vi "Enqueue with Error.vi"(8 "error in (no error)":errorcluster, 10 "Command to Queue":string, 11 "queue in":refnum<queue>) -> (0 "error out":errorcluster, 3 "queue out":refnum<queue>)   [LabVIEW 2010]
doc: "This VI enqueues a command (string) into the input queue. In addition, if any errors are present on the error cluster, the Error state is queued before the input command to be executed in the Error case. Once the error state is queued, the error cluster is cleared and normal operation continues.\n\nInputs:\nqueue in - input queue reference (string queue)\ncommand to queue - command/state to queue (string)\nerror in - error input cluster\n\nOutputs:\nqueue out - referece to input queue (dup)\nerror out - error output cluster"
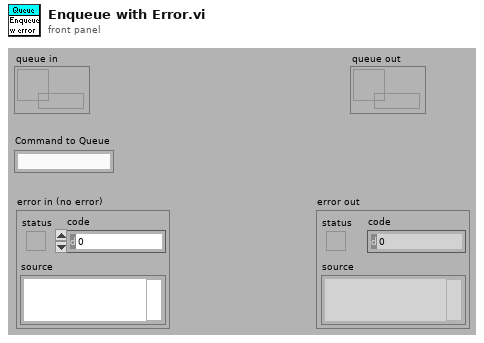
[diagram p1: front panel]
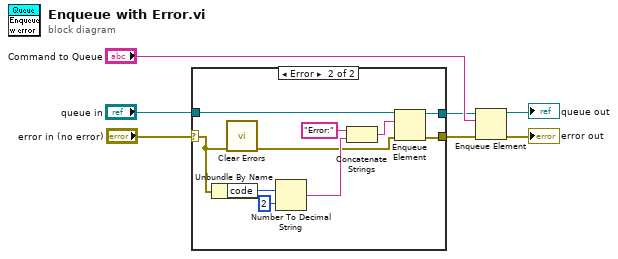
[diagram p0: block diagram]
diagram:
  n1 = case shown="Error" "error in (no error)" {
    selector: "error in (no error)" -> [w8 w12]
    tunnel: [w8 w19] -> w3
    tunnel: "queue in" -> [w9 w17]
    tunnel: [w9 w18] -> w1
    frame No Error {
    }
    frame Error {
      n2 = Unbundle By Name(w12) -> ("code"=w16:i32)
      n3 = call <vilib>:"Clear Errors.vi"("error in (no error)"=w12) -> ("error out"=w11:errorcluster)  [unwired: 6 in]
      n4 = Number To Decimal String(number=w16, width (-)=i16 2) -> (decimal integer string=w13:string)
      n5 = Concatenate Strings("Error:" ("string"), w13) -> (w14:string)
      n6 = Enqueue Element(queue=w17, element=w14, error in (no error)=w11) -> (queue out=w18:refnum<queue>, error out=w19:errorcluster)  [unwired: 1 in, 1 out]
    }
  }
  n7 = Enqueue Element(queue=w1, element="Command to Queue", error in (no error)=w3) -> (queue out=→"queue out":refnum<queue>, error out=→"error out":errorcluster)  [unwired: 1 in, 1 out]
